vi "sv_Check for Frequency Change [Third Octave].vi"(7 "reset filter (F)":bool, 8 "error in (no error)":errorcluster, 9 "frequency range (1/3)":T1={"low band"=enum."20 Hz", "high band"=enum."20000 Hz"}) -> (0 "error out":errorcluster, 2 "Param_has_changed":bool)   [LabVIEW 2017, in "SoundVib_Octave_2014 standard.lvlib"]
uses:
  <vilib>/addons/Sound and Vibration/svt_Octave/SoundVib_Octave_2014 standard.lvlib
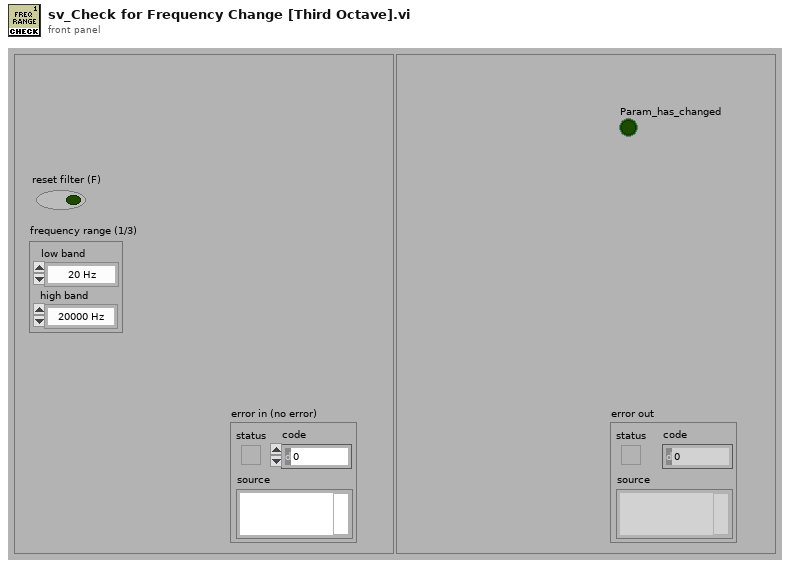
[diagram p1: front panel]
types:
  T1 = cluster{"low band":enum16{"20 Hz", "25 Hz", "31.5 Hz", "40 Hz", "50 Hz", "63 Hz", "80 Hz", "100 Hz", "125 Hz", "160 Hz", "200 Hz", "250 Hz", "315 Hz", "400 Hz", "500 Hz", "630 Hz", "800 Hz", "1000 Hz", "1250 Hz", "1600 Hz", "2000 Hz", "2500 Hz", "3150 Hz", "4000 Hz", "5000 Hz", "6300 Hz", "8000 Hz", "10000 Hz", "12500 Hz", "16000 Hz", "20000 Hz"}, "high band":enum16{"20 Hz", "25 Hz", "31.5 Hz", "40 Hz", "50 Hz", "63 Hz", "80 Hz", "100 Hz", "125 Hz", "160 Hz", "200 Hz", "250 Hz", "315 Hz", "400 Hz", "500 Hz", "630 Hz", "800 Hz", "1000 Hz", "1250 Hz", "1600 Hz", "2000 Hz", "2500 Hz", "3150 Hz", "4000 Hz", "5000 Hz", "6300 Hz", "8000 Hz", "10000 Hz", "12500 Hz", "16000 Hz", "20000 Hz"}}
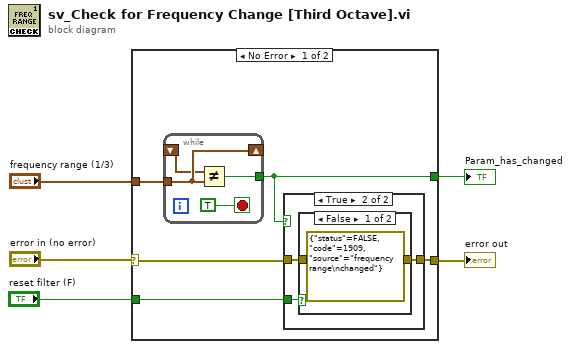
[diagram p0: block diagram]
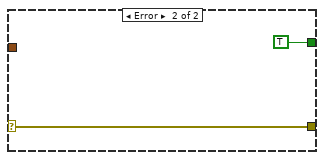
[diagram p4: hidden frame]
diagram:
  n1 = case shown="No Error" "error in (no error)" {
    selector: "error in (no error)" -> [w9 w22]
    tunnel: "frequency range (1/3)" -> [w10 _]
    tunnel: [w7 TRUE] -> w4
    tunnel: [w8 w22] -> w2
    tunnel: "reset filter (F)" -> [w6 _]
    frame No Error {
      n2 = while {
        tunnel: w10 -> [w12]
        tunnel: [w13] -> w7
        shift-left: _ -> [w11]
        shift-right: [w12] -> _
        stop <- TRUE stop-if-true
        n3 = Not Equal?(x=w11, y=w12) -> (x != y?=w13:bool)
      }
      n4 = case shown="True" w7 {
        tunnel: w9 -> [w15 w16]
        tunnel: [w15 w18] -> w8
        tunnel: w6 -> [_ w17]
        frame False {
        }
        frame True {
          n5 = case shown="False" w17 {
            tunnel: [errorcluster {"status"=FALSE, "code"=1909, "source"="frequency range\nchanged"} ("error IO") w20] -> w18
            tunnel: w16 -> [_ w20]
            frame False {
            }
            frame True {
            }
          }
        }
      }
    }
    frame Error {
    }
  }
  "error out" <- w2
  "Param_has_changed" <- w4
